vi "Read Counter Output PWM Module.vi"   [LabVIEW 2020, in "Scan Engine Scripting.lvlib"]
doc: "Returns the channel settings of a counter output PWM module that can be edited and then used to create a new module instance to set into a slot."
uses:
  Scan Engine Scripting.lvlib
  Modules/NI 9474/NI 9474.lvclass
  Modules/NI 9475/NI 9475.lvclass
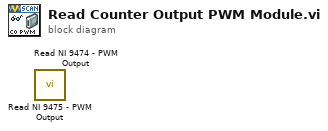
[diagram p0: block diagram]
diagram:
  n1 = call "Read NI 9475 - PWM Output.vi"() -> ()  [unwired: 9 in, 3 out]
  n2 = call "Read NI 9474 - PWM Output.vi"() -> ()  [unwired: 9 in, 3 out]
